vi "AFG3352XGUI.update simple listbox.vi"(0 "listbox":refnum<vi>, 1 "actFrequency":T1, 2 "actAmplitude":T1, 3 "actPhase":T1, 4 "actOffset":T1, 5 "error in (no error)":errorcluster, 7 "actMode":T1, 9 "actBurstMode":T1) -> (19 "error out":errorcluster)   [LabVIEW 2014, in "AFG3352XGUI.lvlib"]
doc: "Displays data of the PowerSupply in advance mode."
uses:
  AFG3352XGUI.lvlib
  CSlibraries-extern/DimLVEvent/DimIndicators/DimIndicators.numericType.ctl
  CSlibraries/UtilityLib/UtilityLib.lvlib
  CSCore/CSSystem/CoreLib/CoreLib.lvlib
  CSlibraries-extern/DimLVEvent/DimIndicators/DimIndicators.lvlib
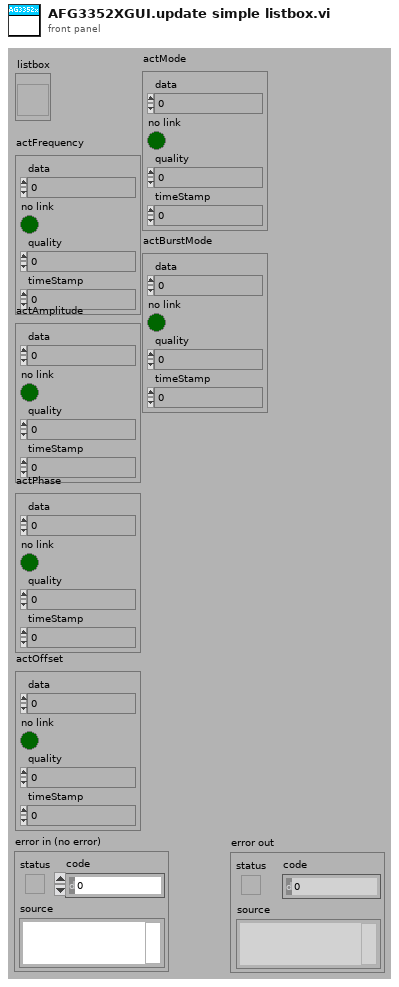
[diagram p1: front panel]
types:
  T1 = typedef "DimIndicators.lvlib/DimIndicators.numericType.ctl" = cluster{"data":dbl, "no link":bool, "quality":i32, "timeStamp":dbl}
  T2 = typedef "UtilityLib.lvlib/UtilityLib.valueStatus.ctl" = enum16{"no info available", "stand by/off", "on", "warning", "alarm/malfunction", "not implemented", "user action required", "important information", "system default", "control default", "indicator default", "button default"}
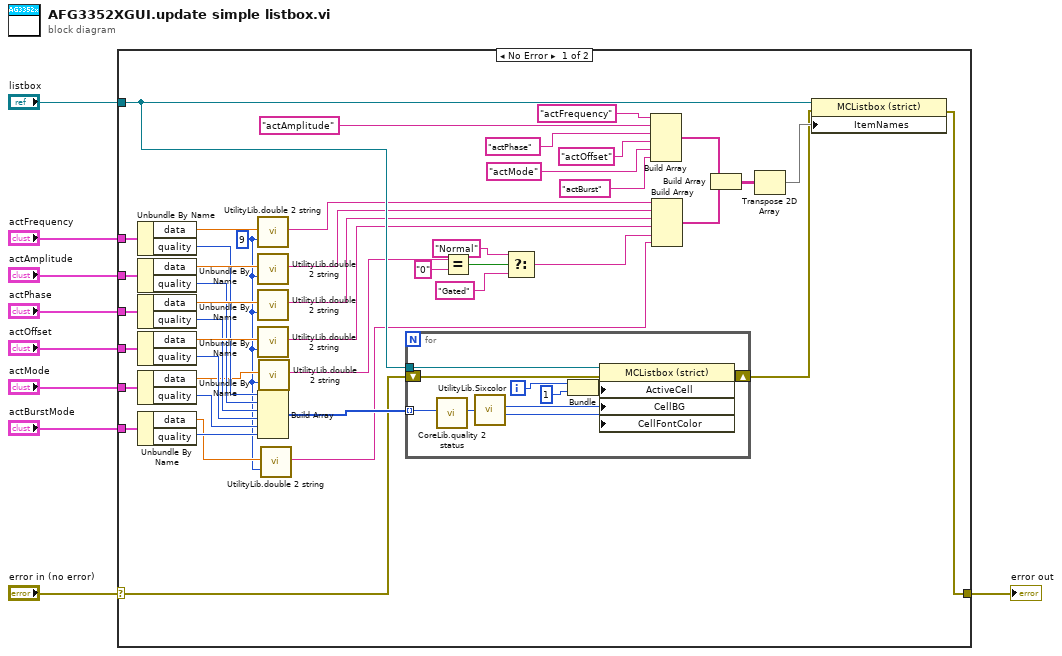
[diagram p0: block diagram]
diagram:
  n1 = case shown="No Error" "error in (no error)" {
    selector: "error in (no error)" -> [w28 w65]
    tunnel: [w26 w65] -> w8
    tunnel: "actFrequency" -> [w41 _]
    tunnel: "actAmplitude" -> [w40 _]
    tunnel: "listbox" -> [w54 _]
    tunnel: "actPhase" -> [w39 _]
    tunnel: "actOffset" -> [w38 _]
    tunnel: "actMode" -> [w25 _]
    tunnel: "actBurstMode" -> [w15 _]
    frame No Error {
      w12 = u8 9 ("length")
      n2 = Unbundle By Name(w41) -> ("data"=w37:dbl, "quality"=w33:i32)
      n3 = Unbundle By Name(w40) -> ("data"=w36:dbl, "quality"=w32:i32)
      n4 = Unbundle By Name(w39) -> ("data"=w35:dbl, "quality"=w31:i32)
      n5 = Unbundle By Name(w38) -> ("data"=w34:dbl, "quality"=w30:i32)
      n6 = Unbundle By Name(w25) -> ("data"=w23:dbl, "quality"=w24:i32)
      n7 = Unbundle By Name(w15) -> ("data"=w13:dbl, "quality"=w14:i32)
      n8 = call "UtilityLib.double 2 string.vi"("Numeric"=w37, "length"=w12) -> ("String"=w53:string)  [unwired: 16 in, 1 out]
      n9 = call "UtilityLib.double 2 string.vi"("Numeric"=w36, "length"=w12) -> ("String"=w52:string)  [unwired: 16 in, 1 out]
      n10 = call "UtilityLib.double 2 string.vi"("Numeric"=w35, "length"=w12) -> ("String"=w51:string)  [unwired: 16 in, 1 out]
      n11 = call "UtilityLib.double 2 string.vi"("Numeric"=w34, "length"=w12) -> ("String"=w50:string)  [unwired: 16 in, 1 out]
      n12 = Build Array(w33, w32, w31, w30, w24, w14) -> (w29:i32[])
      n13 = call "UtilityLib.double 2 string.vi"("Numeric"=w23, "length"=w12) -> ("String"=w21:string)  [unwired: 16 in, 1 out]
      n14 = call "UtilityLib.double 2 string.vi"("Numeric"=w13, "length"=w12) -> ("String"=w10:string)  [unwired: 16 in, 1 out]
      n15 = for {
        tunnel: w54 -> [w64]
        tunnel: w29 -> [w60] mode=indexing
        shift-right: [w55] -> w27
        shift-left: w28 -> [w56]
        i -> [w61]
        n16 = call "CoreLib.quality 2 status.vi"("quality"=w60) -> ("valueStatus"=w59:T2)  [unwired: 18 in]
        n17 = call "UtilityLib.Sixcolor.vi"("State"=w59) -> ("elementBackground"=w58:u32, "elementText"=w57:u32)  [unwired: 2 in, 2 out]
        n18 = Bundle(w61, 1) -> (w63:cluster{i32, i32})  [unwired: 1 in]
        n19 = property on="Property Node" class="MCListbox (strict)"(reference=w64, error in=w56, "ActiveCell"=w63, "CellBG"=w58, "CellFontColor"=w57) -> (error out=w55:errorcluster)  [unwired: 1 out]
      }
      n20 = Equal?(x=w21, y="0") -> (x = y?=w19:bool)
      n21 = Select(t="Normal" ("y"), s=w19, f="Gated") -> (s? t:f=w16:string)
      n22 = Build Array("actFrequency" ("element"), "actAmplitude", "actPhase" ("element"), "actOffset" ("element"), "actMode" ("element"), "actBurst" ("element")) -> (w46:string[])
      n23 = Build Array(w53, w52, w51, w50, w16, w10) -> (w45:string[])
      n24 = Build Array(w46, w45) -> (w44:string[][])
      n25 = Transpose 2D Array(2D array=w44) -> (transposed array=w43:string[][])
      n26 = property on="Property Node" class="MCListbox (strict)"(reference=w54, error in=w27, "ItemNames"=w43) -> (error out=w26:errorcluster)  [unwired: 1 out]
    }
    frame Error {
    }
  }
  "error out" <- w8
